vi "Histogram Window.vi"() -> ()   [LabVIEW 2019, in "Histogram Window.lvlib"]
uses:
  Histogram Window.lvlib
  Histogram Window Q Element v2.ctl
  Histogram Window Q Action v2.ctl
  Updated Plot Info.ctl
  Plot Style 3.ctl
  Fit Plot Request Information.ctl
  <vilib>/Utility/miscctls.llb/LVPointDoubleTypeDef.ctl
  Fit Models.ctl
  <vilib>/Utility/miscctls.llb/LVPoint32TypeDef.ctl
  Plot Histogram.ctl
  Fit Settings.ctl
  <vilib>/Analysis/6fits.llb/Curve Fitting Criteria.ctl
  Ramp Type.ctl
  XY Graph Add-Ons.lvlib
  Notebook.lvlib
  Rich Text Box.lvlib
  <vilib>/Analysis/NI_AALPro.lvlib
  Plot Editor.lvlib
panel:
  out "Histogram Graph TipStrip":string caption="Histogram TipStrip"
  out "Histogram Graph":cluster{"Axis":dbl[], "Histogram":dbl[]}[](graph)
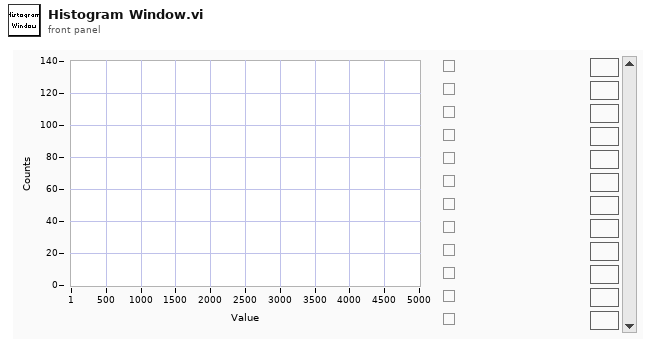
[diagram p1: front panel]
types:
  T1 = typedef "Histogram Window.lvlib/Histogram Window Q Element v2.ctl" = cluster{"Histogram Window Q Action":T2, "Data":variant}
  T2 = typedef "Histogram Window.lvlib/Histogram Window Q Action v2.ctl" = enum16{"Initialization", "Add Histogram", "Delete Histogram", "Delete Selected Histograms", "Clear Graph", "Change Bin Size", "Invert Histogram", "Update Graph", "Edit Plot", "Plot Fit", "Export XYGraph to Notebook", "Select All Plots", "Deselect All Plots", "Invert Plots Selection", "Set Style of Selected Plots", "Save Plot", "Save Selected Plots", "Save All Plots", "Quit"}
  T3 = cluster{"Event Registration Refnum":refnum<event-registration>}
  T4 = typedef "Histogram Window.lvlib/Updated Plot Info.ctl" = cluster{"Plot Index":i32, "Plot Name":string, "# Plots":i32, "Plot Style":T5}
  T5 = typedef "Plot Style 3.ctl" = cluster{"Plot Style":enum16{"unchanged", "Line", "Symbol", "Line + Symbol", "Histogram", "Histogram + Symbol"}, "Histogram Type":enum16{"unchanged", "Left Bound", "Center", "Right Bound"}, "Line Tickness":enum16{"unchanged", "Thin", "1 pixel", "2 pixel", "3 pixel", "4 pixel", "5 pixel"}, "Line Style":enum16{"unchanged", "Plain", "Long Dash", "Short Dash", "Long-Short Dash", "Long-Short-Short Dash"}, "Point Style":enum16{"unchanged", "None", "Empty Circle", "Filled Circle", "Thick Circle", "Dotted Circle", "Empty Square", "Filled Square", "Thick Square", "Dotted Square", "Small Filled Square", "Dot", "Cross", "Tiny Cross", "Large X", "Small x", "Diamond", "Small Empty Square"}, "Line Color":u32, "Point Color":u32, "Anti-aliased":bool, "Line Color Chooser":enum16{"unchanged", "Color Box", "Color List"}, "Point Color Chooser":enum16{"unchanged", "Color Box", "Color List"}, "Line Color List":string, "Point Color List":string}
  T6 = typedef "Histogram Window.lvlib/Plot Histogram.ctl" = cluster{"Plot Name":string, "Histogram":cluster{"Axis":dbl[], "Histogram":dbl[]}, "Plot Style":T5}
  T7 = typedef "LVPoint32TypeDef.ctl" = cluster{"Horizontal":i32, "Vertical":i32}
  T8 = typedef "Fit Plot Request Information.ctl" = cluster{"XY Graph Ref":refnum<vi>, "Mouse Coordinates":T9, "Fit Model":T10, "Plot Index":i32}
  T9 = typedef "LVPointDoubleTypeDef.ctl" = cluster{"X":dbl, "Y":dbl}
  T10 = typedef "Fit Models.ctl" = enum16{"Select a Fit Model...", "           Single Peak", "Gaussian", "Asymmetric Gaussian", "Lorentzian", "Asymmetric Lorentzian", "Gaussian/Lorentzian", "Lorentzian/Gaussian", "           Double Peak", "Two Gaussians", "Two Asymmetric Gaussians", "Two H-Connected Gaussians", "Two T-Connected Gaussians", "Two H-Connected Asymmetric Gaussians", "Two T-Connected Asymmetric Gaussians", "           Triple Peak", "Three Gaussians", "Three Asymmetric Gaussians", "              Decays", "Single Exponential", "Two Exponentials", "               ACF", "2D Gaussian ACF", "2D Gaussian + Blinking ACF", "2D Gaussian + Flow ACF", "3D Gaussian ACF", "3D Gaussian + Blinking ACF", "             Multiplot", "2D Gaussian ACF & 2D Gaussian + Flow ACF"}
  T11 = typedef "Fit Settings.ctl" = cluster{"Use Histogram # Points":bool, "# Fit Plot Points":u32, "Fit Method":T12, "Weighted Histogram Fit":bool, "Show All Fit Components":bool, "Ramp Type":T13}
  T12 = typedef "NI_AALPro.lvlib/Curve Fitting Criteria.ctl" = u16
  T13 = typedef "Ramp Type.ctl" = u16
  T14 = cluster{"CtlRef":refnum<vi>, "Select All Plots":bool}
  T15 = typedef "XY Graph Add-Ons.lvlib/XY Graph Refnum.ctl" = refnum<vi>
  T16 = typedef "D-Only Fixed Parameters.ctl" = cluster{"Fix D-only Peak Location":bool, "Peak Location":dbl, "Fix D-only Peak FWHM":bool, "Peak FWHM":dbl}
  T17 = typedef "Rich Text Box.lvlib/Text Formatting.ctl" = cluster{"Font":string, "Text Color":T18, "Text Background Color":T18, "Text Style":enum16{"Regular", "Bold", "Italic", "Underline", "Strikeout"}, "Font Size (Points)":dbl, "Text Alignment":i32}
  T18 = typedef "Rich Text Box.lvlib/Text Colors.ctl" = enum16{"Unchanged", "Black", "Blue", "Gray", "Green", "Red", "White"}
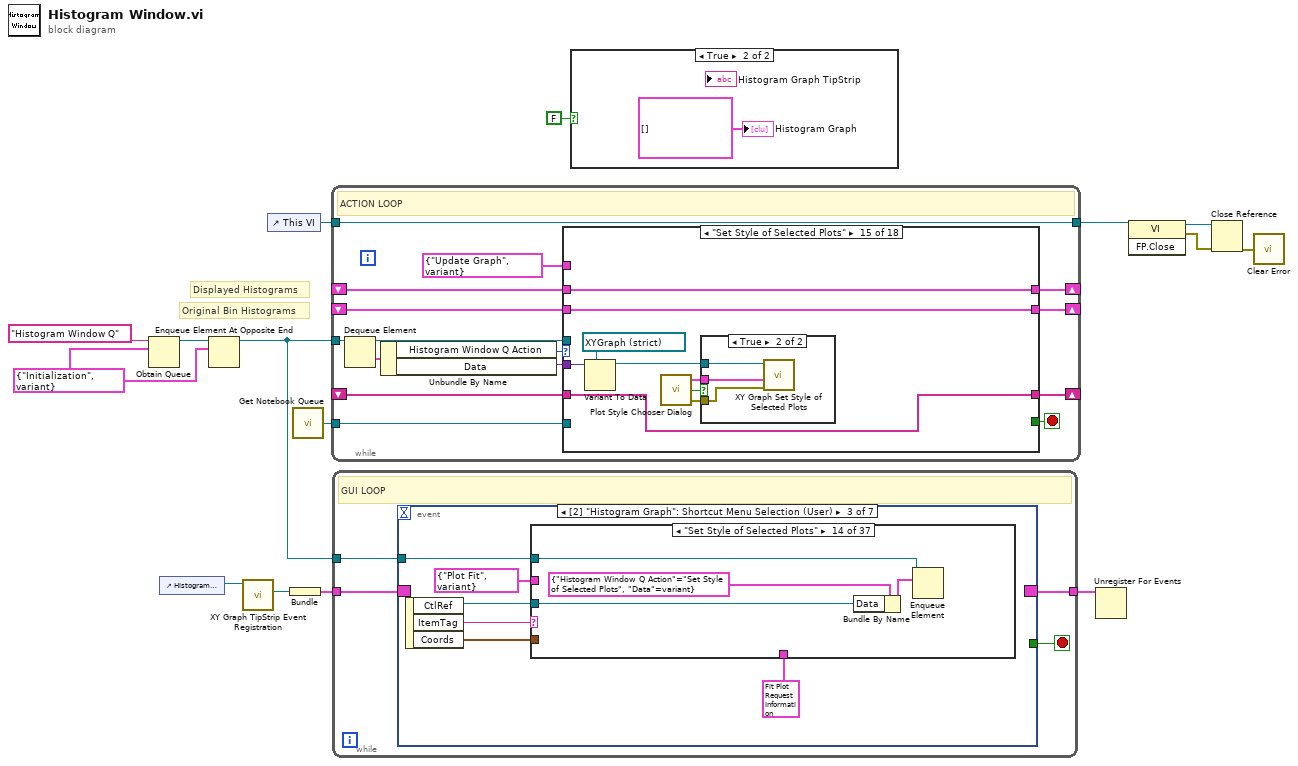
[diagram p0: block diagram]
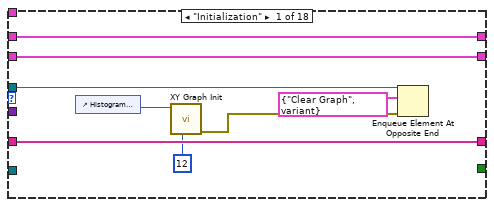
[diagram p3: hidden frame]
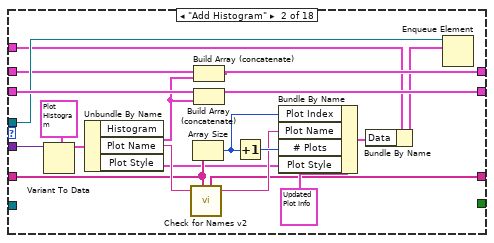
[diagram p4: hidden frame]
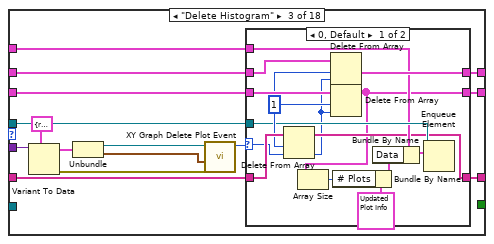
[diagram p5: hidden frame]
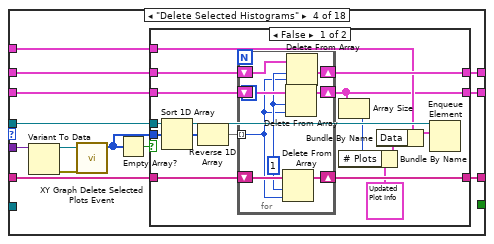
[diagram p7: hidden frame]
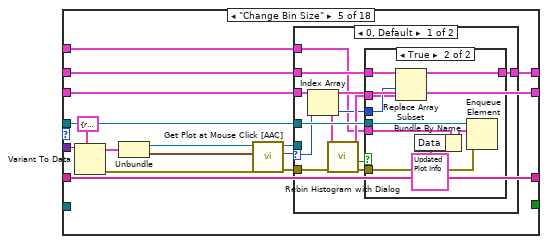
[diagram p9: hidden frame]
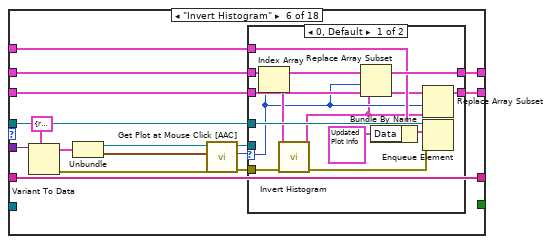
[diagram p12: hidden frame]
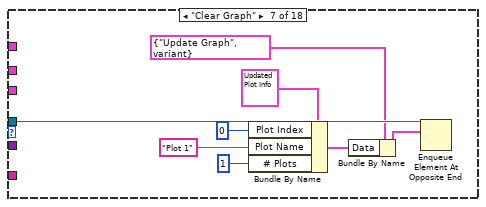
[diagram p14: hidden frame]
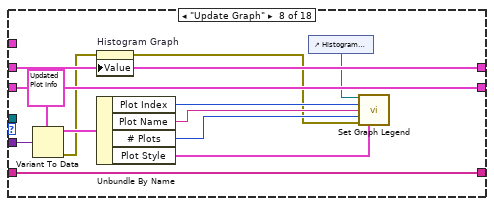
[diagram p15: hidden frame]
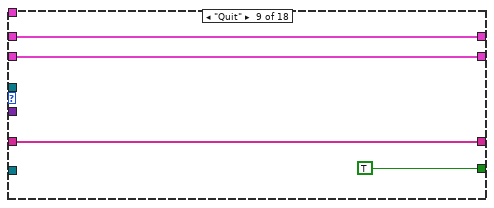
[diagram p16: hidden frame]
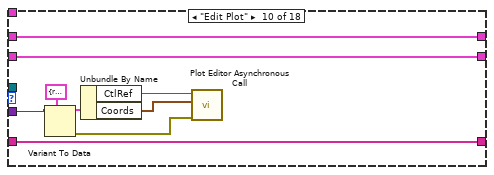
[diagram p17: hidden frame]
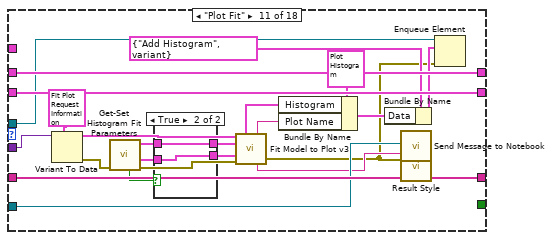
[diagram p18: hidden frame]
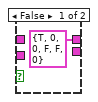
[diagram p19: hidden frame]
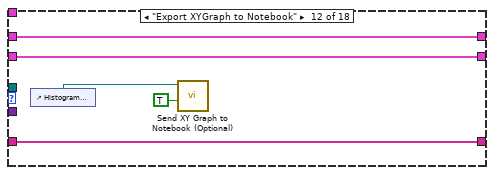
[diagram p20: hidden frame]
diagram:
  w10 = T1 {"Histogram Window Q Action"=enum."Initialization", "Data"=variant} ("ALEX TT Histogram Q Element")
  # "Displayed Histograms"
  # "Original Bin Histograms"
  n1 = Obtain Queue(name (unnamed)="Histogram Window Q", element data type=w10) -> (queue out=w14:refnum<queue>)  [unwired: 3 in, 2 out]
  n2 = control-ref of="Histogram Graph"() -> (w4:refnum<vi>)
  n3 = Enqueue Element At Opposite End(queue=w14, element=w10) -> (queue out=w11:refnum<queue>)  [unwired: 2 in, 2 out]
  n4 = call "XY Graph TipStrip Event Registration.vi"("XY Graph Refnum"=w4) -> ("Event Registration Refnum"=w3:refnum<event-registration>)  [unwired: 8 in, 2 out]
  n5 = control-ref of="This VI"() -> (w6:refnum<vi>)
  n6 = Bundle("Event Registration Refnum"=w3) -> (w8:T3)  [unwired: 1 in]
  n7 = call "Get Notebook Queue.vi"() -> ("Notebook Queue"=w9:refnum<queue>)  [unwired: 9 in]
  n8 = while {
    tunnel: w11 -> [w30]
    shift-right: [w24] -> _
    shift-left: _ -> [w25]
    shift-right: [w22] -> _
    shift-left: _ -> [w23]
    shift-right: [w19] -> _
    shift-left: _ -> [w20]
    tunnel: w9 -> [w17]
    tunnel: w6 -> [w16]
    tunnel: [w16] -> w5
    stop <- w27 stop-if-true
    # "ACTION LOOP"
    n9 = Dequeue Element(queue=w30) -> (queue out=w21:refnum<queue>, element=w29:T1)  [unwired: 2 in, 2 out]
    n10 = Unbundle By Name(w29) -> ("Histogram Window Q Action"=w28:T2, "Data"=w26:variant)
    n11 = case shown="\"Set Style of Selected Plots\"" w28 {
      tunnel: [_ _ _ _ _ _ _ _ TRUE _ _ _ _ _ _ _ _ _] -> w27
      tunnel: w26 -> [_ w57 w73 w103 w144 w182 _ w215 _ w223 w255 _ w266 w275 w282 w301 w313 w324]
      tunnel: w25 -> [w35 w40 w66 w100 w139 w177 _ w218 w219 w231 w247 w261 w272 w278 w279 w308 w319 w330]
      tunnel: [w35 w41 w65 w99 w139 w177 _ w218 w219 w231 w247 w261 w272 w278 w279 w308 w319 w330] -> w24
      tunnel: w23 -> [w36 w58 w68 w102 w133 w168 _ w217 w220 w230 w253 w262 w271 w277 w287 w307 w318 w329]
      tunnel: [w36 w54 w67 w101 w133 w167 _ w217 w220 w230 w253 w262 w271 w277 w287 w307 w318 w329] -> w22
      tunnel: w21 -> [w38 w52 w63 w98 w134 w172 w205 _ _ _ w252 _ _ _ _ _ _ _]
      tunnel: w20 -> [w37 w51 w62 w97 w132 w171 _ w216 w221 w229 w254 w263 w270 w276 w286 w306 w317 w328]
      tunnel: [w37 w49 w61 w96 w131 w170 _ w216 w221 w229 w254 w263 w270 w276 w286 w306 w317 w328] -> w19
      tunnel: T1 {"Histogram Window Q Action"=enum."Update Graph", "Data"=variant} ("ALEX TT Histogram Q Element") -> [_ w45 w60 w95 w130 w169 _ _ _ _ _ _ _ _ _ _ _ _]
      tunnel: w17 -> [_ _ _ _ _ _ _ _ _ _ w243 _ _ _ _ w299 w311 w322]
      frame "Initialization" {
        n12 = control-ref of="Histogram Graph"() -> (w31:refnum<vi>)
        n13 = call "XY Graph Init.vi"("Max Legend Size (8)"=12 ("32bit integer"), "XYGraph in"=w31) -> ("Error Out"=w33:errorcluster)  [unwired: 9 in]
        n14 = Enqueue Element At Opposite End(queue=w38, element=T1 {"Histogram Window Q Action"=enum."Clear Graph", "Data"=variant}, error in (no error)=w33) -> ()  [unwired: 1 in, 3 out]
      }
      frame "Add Histogram" {
        n15 = Variant To Data(type=T6 {"Plot Name"="", "Histogram"={"Axis"=[], "Histogram"=[]}, "Plot Style"={"Plot Style"=enum."Histogram + Symbol", "Histogram Type"=enum."Right Bound", "Line Tickness"=enum."unchanged", "Line Style"=enum."unchanged", "Point Style"=enum."unchanged", "Line Color"=0, "Point Color"=0, "Anti-aliased"=FALSE, "Line Color Chooser"=enum."unchanged", "Point Color Chooser"=enum."unchanged", "Line Color List"="", "Point Color List"=""}} ("output cluster"), Variant=w57) -> (data=w55:T6)  [unwired: 1 in, 1 out]
        n16 = Unbundle By Name(w55) -> ("Histogram"=w50:cluster{"Axis":dbl[], "Histogram":dbl[]}, "Plot Name"=w43:string, "Plot Style"=w39:T5)
        n17 = call "Check for Names v2.vi"("New Name"=w43, "Name List"=w40) -> ("New Name List"=w41:string[], "New Name"=w42:string)  [unwired: 4 in, 2 out]
        n18 = Array Size(array=w40) -> (size(s)=w48:i32)
        n19 = Build Array (concatenate)(w51, w50) -> (w49:cluster{"Axis":dbl[], "Histogram":dbl[]}[])
        n20 = Build Array (concatenate)(w58, w50) -> (w54:cluster{"Axis":dbl[], "Histogram":dbl[]}[])
        n21 = Increment(x=w48) -> (x+1=w53:i32)
        n22 = Bundle By Name(cluster=T4 {"Plot Index"=0, "Plot Name"="", "# Plots"=0, "Plot Style"={"Plot Style"=enum."Line + Symbol", "Histogram Type"=enum."Right Bound", "Line Tickness"=enum."Thin", "Line Style"=enum."unchanged", "Point Style"=enum."unchanged", "Line Color"=0, "Point Color"=0, "Anti-aliased"=FALSE, "Line Color Chooser"=enum."unchanged", "Point Color Chooser"=enum."unchanged", "Line Color List"="", "Point Color List"=""}} ("output cluster"), "Plot Index"=w48, "Plot Name"=w42, "# Plots"=w53, "Plot Style"=w39) -> (w46:T4)
        n23 = Bundle By Name(cluster=w45, "Data"=w46) -> (w47:T1)
        n24 = Enqueue Element(queue=w52, element=w47) -> ()  [unwired: 2 in, 3 out]
      }
      frame "Delete Histogram" {
        n25 = Variant To Data(type=cluster{"CtlRef":refnum<vi>, "Coords":T7} {"CtlRef"=refnum, "Coords"={"Horizontal"=0, "Vertical"=0}} ("output cluster"), Variant=w73) -> (data=w72:cluster{"CtlRef":refnum<vi>, "Coords":T7}, error out=w64:errorcluster)  [unwired: 1 in]
        n26 = Unbundle(w72) -> ("CtlRef"=w70:refnum<vi>, "Coords"=w69:T7)
        n27 = call "XY Graph Delete Plot Event.vi"("Error In"=w64, "Mouse Click Coordinates"=w69, "XYGraph Ref"=w70) -> ("Deleted Plot Index"=w59:i32)  [unwired: 4 in, 4 out]
        n28 = case shown="0, Default" w59 {
          selector: w59 -> [w76 _]
          tunnel: w68 -> [w87 w90]
          tunnel: [w74 w90] -> w67
          tunnel: w66 -> [w86 w89]
          tunnel: [w79 w89] -> w65
          tunnel: w63 -> [w82 _]
          tunnel: w62 -> [w85 w88]
          tunnel: [w84 w88] -> w61
          tunnel: w60 -> [w80 _]
          frame 0, Default {
            w83 = 1 ("length")
            n29 = Delete From Array(array=w86, length=w83, index=w76) -> (array with subset deleted=w79:string[])  [unwired: 1 out]
            n30 = Delete From Array(array=w85, length=w83, index=w76) -> (array with subset deleted=w84:cluster{"Axis":dbl[], "Histogram":dbl[]}[])  [unwired: 1 out]
            n31 = Delete From Array(array=w87, length=w83, index=w76) -> (array with subset deleted=w74:cluster{"Axis":dbl[], "Histogram":dbl[]}[])  [unwired: 1 out]
            n32 = Array Size(array=w74) -> (size(s)=w75:i32)
            n33 = Bundle By Name(cluster=T4 {"Plot Index"=-1, "Plot Name"="", "# Plots"=0, "Plot Style"={"Plot Style"=enum."Histogram + Symbol", "Histogram Type"=enum."Right Bound", "Line Tickness"=enum."unchanged", "Line Style"=enum."unchanged", "Point Style"=enum."unchanged", "Line Color"=0, "Point Color"=0, "Anti-aliased"=FALSE, "Line Color Chooser"=enum."unchanged", "Point Color Chooser"=enum."unchanged", "Line Color List"="", "Point Color List"=""}} ("output cluster"), "# Plots"=w75) -> (w78:T4)
            n34 = Bundle By Name(cluster=w80, "Data"=w78) -> (w81:T1)
            n35 = Enqueue Element(queue=w82, element=w81) -> ()  [unwired: 2 in, 3 out]
          }
          frame -1 {
          }
        }
      }
      frame "Delete Selected Histograms" {
        n36 = Variant To Data(Variant=w103) -> (data=w93:T15, error out=w94:errorcluster)  [unwired: 2 in]
        n37 = call "XY Graph Delete Selected Plots Event.vi"("Error In"=w94, "XYGraph Ref"=w93) -> ("Deleted Plot Indices"=w91:i32[])  [unwired: 5 in, 4 out]
        n38 = Empty Array?(array=w91) -> (empty?=w92:bool)
        n39 = case shown="False" w92 {
          tunnel: w102 -> [w118 w129]
          tunnel: [w107 w129] -> w101
          tunnel: w100 -> [w117 w128]
          tunnel: [w111 w128] -> w99
          tunnel: w98 -> [w114 _]
          tunnel: w97 -> [w116 w127]
          tunnel: [w115 w127] -> w96
          tunnel: w95 -> [w112 _]
          tunnel: w91 -> [w106 _]
          frame False {
            n40 = Sort 1D Array(array=w106) -> (sorted array=w105:i32[])
            n41 = Reverse 1D Array(array=w105) -> (reversed array=w104:i32[])
            n42 = for {
              shift-right: [w123] -> w115
              shift-left: w116 -> [w124]
              shift-right: [w120] -> w107
              shift-left: w118 -> [w126]
              shift-right: [w121] -> w111
              shift-left: w117 -> [w125]
              tunnel: w104 -> [w119] mode=indexing
              w122 = 1 ("length")
              n43 = Delete From Array(array=w125, length=w122, index=w119) -> (array with subset deleted=w121:string[])  [unwired: 1 out]
              n44 = Delete From Array(array=w126, length=w122, index=w119) -> (array with subset deleted=w120:cluster{"Axis":dbl[], "Histogram":dbl[]}[])  [unwired: 1 out]
              n45 = Delete From Array(array=w124, length=w122, index=w119) -> (array with subset deleted=w123:cluster{"Axis":dbl[], "Histogram":dbl[]}[])  [unwired: 1 out]
            }
            n46 = Array Size(array=w107) -> (size(s)=w108:i32)
            n47 = Bundle By Name(cluster=T4 {"Plot Index"=-1, "Plot Name"="", "# Plots"=0, "Plot Style"={"Plot Style"=enum."Histogram + Symbol", "Histogram Type"=enum."Right Bound", "Line Tickness"=enum."unchanged", "Line Style"=enum."unchanged", "Point Style"=enum."unchanged", "Line Color"=0, "Point Color"=0, "Anti-aliased"=FALSE, "Line Color Chooser"=enum."unchanged", "Point Color Chooser"=enum."unchanged", "Line Color List"="", "Point Color List"=""}} ("output cluster"), "# Plots"=w108) -> (w110:T4)
            n48 = Bundle By Name(cluster=w112, "Data"=w110) -> (w113:T1)
            n49 = Enqueue Element(queue=w114, element=w113) -> ()  [unwired: 2 in, 3 out]
          }
          frame True {
          }
        }
      }
      frame "Change Bin Size" {
        n50 = Variant To Data(type=cluster{"CtlRef":refnum<vi>, "Coords":T7} {"CtlRef"=refnum, "Coords"={"Horizontal"=0, "Vertical"=0}} ("output cluster"), Variant=w144) -> (data=w143:cluster{"CtlRef":refnum<vi>, "Coords":T7}, error out=w138:errorcluster)  [unwired: 1 in]
        n51 = Unbundle(w143) -> ("CtlRef"=w141:refnum<vi>, "Coords"=w140:T7)
        n52 = call "Get Plot at Mouse Click [AAC].vi"("error in (no error)"=w138, "Mouse Click Coordinates"=w140, "XYGraph Ref"=w141) -> ("error out"=w136:errorcluster, "Plot at Coordinates"=w137:i32, "XYGraph Ref"=w135:T15)  [unwired: 2 in, 4 out]
        n53 = case shown="0, Default" w137 {
          selector: w137 -> [w146 _]
          tunnel: w136 -> [w155 _]
          tunnel: w135 -> [_ _]
          tunnel: w134 -> [w154 _]
          tunnel: w133 -> [w152 _]
          tunnel: w132 -> [w149 w166]
          tunnel: [w148 w166] -> w131
          tunnel: w130 -> [w145 _]
          frame 0, Default {
            n54 = Index Array(array=w152, index=w146) -> (element=w151:cluster{"Axis":dbl[], "Histogram":dbl[]})
            n55 = call "Rebin Histogram with Dialog.vi"("error in (no error)"=w155, "Original Bin Histogram"=w151) -> ("error out"=w153:errorcluster, "OK?"=w150:bool, "Rebinned Histogram"=w147:cluster{"Axis":dbl[], "Histogram":dbl[]})  [unwired: 7 in]
            n56 = case shown="True" w150 {
              tunnel: w154 -> [_ w165]
              tunnel: w153 -> [_ w164]
              tunnel: w149 -> [w156 w163]
              tunnel: [w156 w162] -> w148
              tunnel: w147 -> [_ w160]
              tunnel: w146 -> [_ w161]
              tunnel: w145 -> [_ w159]
              frame False {
              }
              frame True {
                n57 = Replace Array Subset(array=w163, new element=w160, index=w161) -> (w162:cluster{"Axis":dbl[], "Histogram":dbl[]}[])
                n58 = Bundle By Name(cluster=w159, "Data"=T4 {"Plot Index"=-1, "Plot Name"="", "# Plots"=0, "Plot Style"={"Plot Style"=enum."Histogram + Symbol", "Histogram Type"=enum."Right Bound", "Line Tickness"=enum."unchanged", "Line Style"=enum."unchanged", "Point Style"=enum."unchanged", "Line Color"=0, "Point Color"=0, "Anti-aliased"=FALSE, "Line Color Chooser"=enum."unchanged", "Point Color Chooser"=enum."unchanged", "Line Color List"="", "Point Color List"=""}} ("Updated Plot Info")) -> (w158:T1)
                n59 = Enqueue Element(queue=w165, element=w158, error in (no error)=w164) -> ()  [unwired: 1 in, 3 out]
              }
            }
          }
          frame -1 {
          }
        }
      }
      frame "Invert Histogram" {
        n60 = Variant To Data(type=cluster{"CtlRef":refnum<vi>, "Coords":T7} {"CtlRef"=refnum, "Coords"={"Horizontal"=0, "Vertical"=0}} ("output cluster"), Variant=w182) -> (data=w181:cluster{"CtlRef":refnum<vi>, "Coords":T7}, error out=w176:errorcluster)  [unwired: 1 in]
        n61 = Unbundle(w181) -> ("CtlRef"=w179:refnum<vi>, "Coords"=w178:T7)
        n62 = call "Get Plot at Mouse Click [AAC].vi"("error in (no error)"=w176, "Mouse Click Coordinates"=w178, "XYGraph Ref"=w179) -> ("error out"=w174:errorcluster, "Plot at Coordinates"=w175:i32, "XYGraph Ref"=w173:T15)  [unwired: 2 in, 4 out]
        n63 = case shown="0, Default" w175 {
          selector: w175 -> [w185 _]
          tunnel: w174 -> [w195 _]
          tunnel: w173 -> [_ _]
          tunnel: w172 -> [w194 _]
          tunnel: w171 -> [w190 w197]
          tunnel: [w192 w197] -> w170
          tunnel: w169 -> [w191 _]
          tunnel: w168 -> [w186 w196]
          tunnel: [w183 w196] -> w167
          frame 0, Default {
            n64 = Index Array(array=w190, index=w185) -> (element=w189:cluster{"Axis":dbl[], "Histogram":dbl[]})
            n65 = call "Invert Histogram.vi"("error in (no error)"=w195, "Histogram"=w189) -> ("error out"=w193:errorcluster, "Inverted Histogram"=w184:cluster{"Axis":dbl[], "Histogram":dbl[]})  [unwired: 8 in]
            n66 = Replace Array Subset(array=w190, new element=w184, index=w185) -> (w192:cluster{"Axis":dbl[], "Histogram":dbl[]}[])
            n67 = Bundle By Name(cluster=w191, "Data"=T4 {"Plot Index"=-1, "Plot Name"="", "# Plots"=0, "Plot Style"={"Plot Style"=enum."Histogram + Symbol", "Histogram Type"=enum."Right Bound", "Line Tickness"=enum."unchanged", "Line Style"=enum."unchanged", "Point Style"=enum."unchanged", "Line Color"=0, "Point Color"=0, "Anti-aliased"=FALSE, "Line Color Chooser"=enum."unchanged", "Point Color Chooser"=enum."unchanged", "Line Color List"="", "Point Color List"=""}} ("output cluster")) -> (w188:T1)
            n68 = Replace Array Subset(array=w186, new element=w184, index=w185) -> (w183:cluster{"Axis":dbl[], "Histogram":dbl[]}[])
            n69 = Enqueue Element(queue=w194, element=w188, error in (no error)=w193) -> ()  [unwired: 1 in, 3 out]
          }
          frame -1 {
          }
        }
      }
      frame "Clear Graph" {
        n70 = Bundle By Name(cluster=T4 {"Plot Index"=0, "Plot Name"="", "# Plots"=0, "Plot Style"={"Plot Style"=enum."Histogram + Symbol", "Histogram Type"=enum."Right Bound", "Line Tickness"=enum."unchanged", "Line Style"=enum."unchanged", "Point Style"=enum."unchanged", "Line Color"=0, "Point Color"=0, "Anti-aliased"=FALSE, "Line Color Chooser"=enum."unchanged", "Point Color Chooser"=enum."unchanged", "Line Color List"="", "Point Color List"=""}} ("output cluster"), "Plot Index"=0, "Plot Name"="Plot 1", "# Plots"=1 ("# Legend Rows")) -> (w201:T4)
        n71 = Bundle By Name(cluster=T1 {"Histogram Window Q Action"=enum."Update Graph", "Data"=variant} ("ALEX TT Histogram Q Element"), "Data"=w201) -> (w203:T1)
        n72 = Enqueue Element At Opposite End(queue=w205, element=w203) -> ()  [unwired: 2 in, 3 out]
      }
      frame "Update Graph" {
        n73 = Variant To Data(type=T4 {"Plot Index"=0, "Plot Name"="", "# Plots"=0, "Plot Style"={"Plot Style"=enum."Histogram + Symbol", "Histogram Type"=enum."Right Bound", "Line Tickness"=enum."unchanged", "Line Style"=enum."unchanged", "Point Style"=enum."unchanged", "Line Color"=0, "Point Color"=0, "Anti-aliased"=FALSE, "Line Color Chooser"=enum."unchanged", "Point Color Chooser"=enum."unchanged", "Line Color List"="", "Point Color List"=""}} ("output cluster"), Variant=w215) -> (data=w213:T4, error out=w208:errorcluster)  [unwired: 1 in]
        n74 = property on="Histogram Graph" class="XYGraph (strict)"(error in=w208, "Value"=w216) -> (error out=w207:errorcluster)  [unwired: 1 in, 1 out]
        n75 = Unbundle By Name(w213) -> ("Plot Index"=w212:i32, "Plot Name"=w210:string, "# Plots"=w211:i32, "Plot Style"=w206:T5)
        n76 = control-ref of="Histogram Graph"() -> (w209:refnum<vi>)
        n77 = call "Set Graph Legend.vi"("XYGraph in"=w209, "Active Plot"=w212, "Plot Name"=w210, "# Plots"=w211, "error in (no error)"=w207, "Plot Style"=w206) -> ()  [unwired: 9 in, 1 out]
      }
      frame "Quit" {
      }
      frame "Edit Plot" {
        n78 = Variant To Data(type=cluster{"CtlRef":refnum<vi>, "Coords":T7} {"CtlRef"=refnum, "Coords"={"Horizontal"=0, "Vertical"=0}} ("output cluster"), Variant=w223) -> (data=w225:cluster{"CtlRef":refnum<vi>, "Coords":T7}, error out=w227:errorcluster)  [unwired: 1 in]
        n79 = Unbundle By Name(w225) -> ("CtlRef"=w228:refnum<vi>, "Coords"=w226:T7)
        n80 = call "Plot Editor Asynchronous Call.vi"("error in (no error)"=w227, "Coords"=w226, "XYGraph in"=w228) -> ()  [unwired: 5 in, 4 out]
      }
      frame "Plot Fit" {
        n81 = Variant To Data(type=T8 {"XY Graph Ref"=refnum, "Mouse Coordinates"={"X"=0.0, "Y"=0.0}, "Fit Model"=enum."Select a Fit Model...", "Plot Index"=-1} ("output cluster"), Variant=w255) -> (data=w240:T8, error out=w238:errorcluster)  [unwired: 1 in]
        n82 = call "Get-Set Histogram Fit Parameters.vi"("Error In"=w238) -> ("Error Out"=w237:errorcluster, "Fixed Parameters"=w232:T16, "Fit Settings"=w235:T11, "Initialized?"=w236:bool)  [unwired: 7 in]
        n83 = case shown="True" w236 {
          tunnel: w235 -> [_ w258]
          tunnel: [T11 {"Use Histogram # Points"=TRUE, "# Fit Plot Points"=0, "Fit Method"=0, "Weighted Histogram Fit"=FALSE, "Show All Fit Components"=FALSE, "Ramp Type"=0} ("Fit Settings") w258] -> w234
          tunnel: [_ w257] -> w233
          tunnel: w232 -> [_ w257]
          frame False {
          }
          frame True {
          }
        }
        n84 = call "Fit Model to Plot v3.vi"("Fit Plot Information"=w240, "Fit Settings"=w234, "Fixed Parameters"=w233, "error in (no error)"=w237) -> ("Fitted Plot"=w245:cluster{"X Array":dbl[], "Y Array":dbl[]}, "Plot Name"=w244:string, "Fit Result String"=w242:string, "error out"=w241:errorcluster)  [unwired: 5 in, 3 out]
        n85 = Bundle By Name(cluster=T6 {"Plot Name"="", "Histogram"={"Axis"=[], "Histogram"=[]}, "Plot Style"={"Plot Style"=enum."Line", "Histogram Type"=enum."Center", "Line Tickness"=enum."2 pixel", "Line Style"=enum."Plain", "Point Style"=enum."None", "Line Color"=16711680, "Point Color"=16711680, "Anti-aliased"=TRUE, "Line Color Chooser"=enum."Color Box", "Point Color Chooser"=enum."Color Box", "Line Color List"="", "Point Color List"=""}} ("output cluster"), "Histogram"=w245, "Plot Name"=w244) -> (w249:T6)
        n86 = Bundle By Name(cluster=T1 {"Histogram Window Q Action"=enum."Add Histogram", "Data"=variant} ("element"), "Data"=w249) -> (w250:T1)
        n87 = call "Result Style.vi"() -> ("Default Text Formatting"=w239:T17)
        n88 = call "Send Message to Notebook.vi"("Notebook Queue"=w243, "Message"=w242, "Error In"=w241, "Text Formatting"=w239) -> ()  [unwired: 15 in, 1 out]
        n89 = Enqueue Element(queue=w252, element=w250, error in (no error)=w241) -> ()  [unwired: 1 in, 3 out]
      }
      frame "Export XYGraph to Notebook" {
        n90 = control-ref of="Histogram Graph"() -> (w260:refnum<vi>)
        n91 = call "Send XY Graph to Notebook (Optional).vi"("Send Graph to Notebook?"=TRUE, "XYGraph in"=w260) -> ()  [unwired: 9 in, 1 out]
      }
      frame "Select All Plots", "Deselect All Plots" {
        n92 = Variant To Data(type=T14 {"CtlRef"=refnum, "Select All Plots"=TRUE} ("output cluster"), Variant=w266) -> (data=w269:T14, error out=w264:errorcluster)  [unwired: 1 in]
        n93 = Unbundle(w269) -> ("CtlRef"=w268:refnum<vi>, "Select All Plots"=w267:bool)
        n94 = call "XY Graph Select All Plots Event.vi"("Error In"=w264, "Select (T)/Deselect"=w267, "XYGraph Ref"=w268) -> ()  [unwired: 5 in, 4 out]
      }
      frame "Invert Plots Selection" {
        n95 = Variant To Data(Variant=w275) -> (data=w274:T15, error out=w273:errorcluster)  [unwired: 2 in]
        n96 = call "XY Graph Invert Plots Selection Event.vi"("Error In"=w273, "XYGraph Ref"=w274) -> ()  [unwired: 6 in, 4 out]
      }
      frame "Set Style of Selected Plots" {
        n97 = Variant To Data(type=refnum<vi> refnum ("XYGraph Ref"), Variant=w282) -> (data=w280:refnum<vi>)  [unwired: 1 in, 1 out]
        n98 = call "Plot Style Chooser Dialog.vi"() -> ("Plot Style out"=w285:T5, "Cancelled?"=w284:bool, "Error Out"=w283:errorcluster)  [unwired: 7 in]
        n99 = case shown="True" w284 {
          tunnel: w280 -> [_ w290]
          tunnel: w285 -> [_ w289]
          tunnel: w283 -> [_ w288]
          frame False {
          }
          frame True {
            n100 = call "XY Graph Set Style of Selected Plots.vi"("Error In"=w288, "Plot Style"=w289, "XYGraph Ref"=w290) -> ()  [unwired: 5 in, 4 out]
          }
        }
      }
      frame "Save Plot" {
        n101 = Variant To Data(type=cluster{"CtlRef":refnum<vi>, "Coords":T7} {"CtlRef"=refnum, "Coords"={"Horizontal"=0, "Vertical"=0}} ("output cluster"), Variant=w301) -> (data=w304:cluster{"CtlRef":refnum<vi>, "Coords":T7}, error out=w300:errorcluster)  [unwired: 1 in]
        n102 = Unbundle By Name(w304) -> ("CtlRef"=w302:refnum<vi>, "Coords"=w303:T7)
        n103 = call "XY Graph Save Plot Event.vi"("Error In"=w300, "Mouse Click Coordinates"=w303, "XYGraph Ref"=w302) -> ("Error Out"=w294:errorcluster, "Message"=w297:string, "File Path"=w291:path, "Plot Name"=w292:string)  [unwired: 3 in, 2 out]
        n104 = Format Into String(format string=" from %s saved as %s", initial string=w297, error in=w294, w292, w291) -> (resulting string=w295:string, error out=w293:errorcluster)
        n105 = call "Message Style.vi"() -> ("Message Formatting"=w298:T17)
        n106 = call "Send Message to Notebook.vi"("Notebook Queue"=w299, "Message"=w295, "Error In"=w293, "Text Formatting"=w298) -> ()  [unwired: 15 in, 1 out]
      }
      frame "Save Selected Plots" {
        n107 = Variant To Data(Variant=w313) -> (data=w316:T15, error out=w314:errorcluster)  [unwired: 2 in]
        n108 = call "XY Graph Save Selected Plots Event.vi"("Error In"=w314, "Save All Plots? (T)"=FALSE, "XYGraph Ref"=w316) -> ("Error Out"=w310:errorcluster, "Message"=w309:string)  [unwired: 3 in, 4 out]
        n109 = call "Message Style.vi"() -> ("Message Formatting"=w312:T17)
        n110 = call "Send Message to Notebook.vi"("Notebook Queue"=w311, "Message"=w309, "Error In"=w310, "Text Formatting"=w312) -> ()  [unwired: 15 in, 1 out]
      }
      frame "Save All Plots" {
        n111 = Variant To Data(Variant=w324) -> (data=w327:T15, error out=w325:errorcluster)  [unwired: 2 in]
        n112 = call "XY Graph Save Selected Plots Event.vi"("Error In"=w325, "Save All Plots? (T)"=TRUE, "XYGraph Ref"=w327) -> ("Error Out"=w321:errorcluster, "Message"=w320:string)  [unwired: 3 in, 4 out]
        n113 = call "Message Style.vi"() -> ("Message Formatting"=w323:T17)
        n114 = call "Send Message to Notebook.vi"("Notebook Queue"=w322, "Message"=w320, "Error In"=w321, "Text Formatting"=w323) -> ()  [unwired: 15 in, 1 out]
      }
    }
  }
  n115 = while {
    tunnel: w11 -> [w333]
    tunnel: w8 -> [w331]
    tunnel: [w332] -> w2
    stop <- w334 stop-if-true
    # "GUI LOOP"
    n116 = event shown="[2] \"Histogram Graph\": Shortcut Menu Selection (User)" {
      selector: w331 -> [_ _ _ _ w557 w562 w563]
      dyn-events: [_ _ _ _ w556 w561 w563] -> w332
      timeout: _ -> [_ _ _ _ _ _ _]
      tunnel: [w337 _ _ _ _ _ _] -> w334
      tunnel: w333 -> [w336 w344 w347 _ _ _ _]
      event Panel Close? {
        w337 = TRUE
        n117 = event-data() -> ()  [unwired: 1 in, 3 out]
        n118 = Enqueue Element(queue=w336, element=T1 {"Histogram Window Q Action"=enum."Quit", "Data"=variant} ("ALEX TT Histogram Q Element")) -> ()  [unwired: 2 in, 3 out]
        n119 = event-data("Discard?"=w337) -> ()  [unwired: 1 in, 1 out]
      }
      event Pane Size {
        n120 = event-data() -> ()  [unwired: 1 in, 1 out]
        n121 = control-ref of="Histogram Graph"() -> (w339:refnum<vi>)
        n122 = call "XY Graph Number of Plots.vi"("XYGraph in"=w339) -> ("# Plots"=w338:i32)  [unwired: 9 in, 1 out]
        n123 = Bundle By Name(cluster=T4 {"Plot Index"=-1, "Plot Name"="", "# Plots"=0, "Plot Style"={"Plot Style"=enum."Histogram + Symbol", "Histogram Type"=enum."Right Bound", "Line Tickness"=enum."unchanged", "Line Style"=enum."unchanged", "Point Style"=enum."unchanged", "Line Color"=0, "Point Color"=0, "Anti-aliased"=FALSE, "Line Color Chooser"=enum."unchanged", "Point Color Chooser"=enum."unchanged", "Line Color List"="", "Point Color List"=""}} ("Updated Plot Info"), "# Plots"=w338) -> (w340:T4)
        n124 = Bundle By Name(cluster=T1 {"Histogram Window Q Action"=enum."Update Graph", "Data"=variant} ("element"), "Data"=w340) -> (w342:T1)
        n125 = Enqueue Element(queue=w344, element=w342) -> ()  [unwired: 2 in, 3 out]
      }
      event "Histogram Graph": Shortcut Menu Selection (User) {
        n126 = event-data() -> ("CtlRef"=w350:refnum<vi>, "ItemTag"=w349:string, "Coords"=w348:T7)  [unwired: 1 in]
        n127 = case shown="\"Set Style of Selected Plots\"" w349 {
          tunnel: w350 -> [_ w353 _ _ w362 w364 w372 w378 w384 w386 w394 w396 w404 w406 w410 w414 _ w424 w432 w440 w448 w456 w464 w472 w480 w488 w496 w504 w512 w520 w528 w536 w544 _ _ w548 w549]
          tunnel: w348 -> [_ w352 _ _ w361 _ w371 w377 w383 _ _ _ _ _ _ _ _ w423 w431 w439 w447 w455 w463 w471 w479 w487 w495 w503 w511 w519 w527 w535 w543 _ _ _ _]
          tunnel: w347 -> [_ w357 _ _ w363 w367 w373 w379 w385 w389 w395 w399 w405 w409 w413 w417 _ w425 w433 w441 w449 w457 w465 w473 w481 w489 w497 w505 w513 w521 w529 w537 w545 w547 _ _ _]
          tunnel: T1 {"Histogram Window Q Action"=enum."Plot Fit", "Data"=variant} ("ALEX TT Histogram Q Element") -> [_ _ _ _ _ _ _ _ _ _ _ _ _ _ _ _ _ w420 w427 w435 w443 w451 w459 w467 w475 w483 w491 w499 w507 w515 w523 w531 w540 _ _ _ _]
          tunnel: T8 {"XY Graph Ref"=refnum, "Mouse Coordinates"={"X"=0.0, "Y"=0.0}, "Fit Model"=enum."Select a Fit Model...", "Plot Index"=-1} ("output cluster") -> [_ _ _ _ _ _ _ _ _ _ _ _ _ _ _ _ _ w418 w426 w434 w442 w450 w458 w466 w474 w482 w490 w498 w506 w514 w522 w530 w539 _ _ _ _]
          frame "", Default {
          }
          frame "Edit Plot" {
            n128 = Bundle By Name(cluster=cluster{"CtlRef":refnum<vi>, "Coords":T7} {"CtlRef"=refnum, "Coords"={"Horizontal"=0, "Vertical"=0}} ("output cluster"), "CtlRef"=w353, "Coords"=w352) -> (w355:cluster{"CtlRef":refnum<vi>, "Coords":T7})
            n129 = Bundle By Name(cluster=T1 {"Histogram Window Q Action"=enum."Edit Plot", "Data"=variant} ("ALEX TT Histogram Q Element"), "Data"=w355) -> (w351:T1)
            n130 = Enqueue Element(queue=w357, element=w351) -> ()  [unwired: 2 in, 3 out]
          }
          frame "Send Plot to Advanced Plot Window" {
          }
          frame "Send Graph to Advanced Plot Window" {
          }
          frame "Delete Plot" {
            n131 = Bundle("CtlRef"=w362, "Coords"=w361) -> (w359:cluster{"CtlRef":refnum<vi>, "Coords":T7})  [unwired: 1 in]
            n132 = Bundle By Name(cluster=T1 {"Histogram Window Q Action"=enum."Delete Histogram", "Data"=variant} ("ALEX TT Histogram Q Element"), "Data"=w359) -> (w360:T1)
            n133 = Enqueue Element(queue=w363, element=w360) -> ()  [unwired: 2 in, 3 out]
          }
          frame "Delete Selected Plots" {
            n134 = Bundle By Name(cluster=T1 {"Histogram Window Q Action"=enum."Delete Selected Histograms", "Data"=variant} ("ALEX TT Histogram Q Element"), "Data"=w364) -> (w366:T1)
            n135 = Enqueue Element(queue=w367, element=w366) -> ()  [unwired: 2 in, 3 out]
          }
          frame "Save Plot" {
            n136 = Bundle("CtlRef"=w372, "Coords"=w371) -> (w369:cluster{"CtlRef":refnum<vi>, "Coords":T7})  [unwired: 1 in]
            n137 = Bundle By Name(cluster=T1 {"Histogram Window Q Action"=enum."Save Plot", "Data"=variant} ("ALEX TT Histogram Q Element"), "Data"=w369) -> (w370:T1)
            n138 = Enqueue Element(queue=w373, element=w370) -> ()  [unwired: 2 in, 3 out]
          }
          frame "Rebin Histogram" {
            n139 = Bundle("CtlRef"=w378, "Coords"=w377) -> (w375:cluster{"CtlRef":refnum<vi>, "Coords":T7})  [unwired: 1 in]
            n140 = Bundle By Name(cluster=T1 {"Histogram Window Q Action"=enum."Change Bin Size", "Data"=variant} ("ALEX TT Histogram Q Element"), "Data"=w375) -> (w376:T1)
            n141 = Enqueue Element(queue=w379, element=w376) -> ()  [unwired: 2 in, 3 out]
          }
          frame "Invert Histogram" {
            n142 = Bundle("CtlRef"=w384, "Coords"=w383) -> (w381:cluster{"CtlRef":refnum<vi>, "Coords":T7})  [unwired: 1 in]
            n143 = Bundle By Name(cluster=T1 {"Histogram Window Q Action"=enum."Invert Histogram", "Data"=variant} ("ALEX TT Histogram Q Element"), "Data"=w381) -> (w382:T1)
            n144 = Enqueue Element(queue=w385, element=w382) -> ()  [unwired: 2 in, 3 out]
          }
          frame "Clear Graph" {
            n145 = Bundle By Name(cluster=T1 {"Histogram Window Q Action"=enum."Clear Graph", "Data"=variant} ("ALEX TT Histogram Q Element"), "Data"=w386) -> (w388:T1)
            n146 = Enqueue Element(queue=w389, element=w388) -> ()  [unwired: 2 in, 3 out]
          }
          frame "Select All Plots" {
            n147 = Bundle("CtlRef"=w394, TRUE) -> (w392:cluster{"CtlRef":refnum<vi>, bool})  [unwired: 1 in]
            n148 = Bundle By Name(cluster=T1 {"Histogram Window Q Action"=enum."Select All Plots", "Data"=variant} ("ALEX TT Histogram Q Element"), "Data"=w392) -> (w393:T1)
            n149 = Enqueue Element(queue=w395, element=w393) -> ()  [unwired: 2 in, 3 out]
          }
          frame "Invert Plots Selection" {
            n150 = Bundle By Name(cluster=T1 {"Histogram Window Q Action"=enum."Invert Plots Selection", "Data"=variant} ("element"), "Data"=w396) -> (w397:T1)
            n151 = Enqueue Element(queue=w399, element=w397) -> ()  [unwired: 2 in, 3 out]
          }
          frame "Deselect All Plots" {
            n152 = Bundle("CtlRef"=w404, FALSE) -> (w402:cluster{"CtlRef":refnum<vi>, bool})  [unwired: 1 in]
            n153 = Bundle By Name(cluster=T1 {"Histogram Window Q Action"=enum."Select All Plots", "Data"=variant} ("ALEX TT Histogram Q Element"), "Data"=w402) -> (w403:T1)
            n154 = Enqueue Element(queue=w405, element=w403) -> ()  [unwired: 2 in, 3 out]
          }
          frame "Set Style of Selected Plots" {
            n155 = Bundle By Name(cluster=T1 {"Histogram Window Q Action"=enum."Set Style of Selected Plots", "Data"=variant} ("ALEX TT Histogram Q Element"), "Data"=w406) -> (w408:T1)
            n156 = Enqueue Element(queue=w409, element=w408) -> ()  [unwired: 2 in, 3 out]
          }
          frame "Save Selected Plots" {
            n157 = Bundle By Name(cluster=T1 {"Histogram Window Q Action"=enum."Save Selected Plots", "Data"=variant} ("ALEX TT Histogram Q Element"), "Data"=w410) -> (w412:T1)
            n158 = Enqueue Element(queue=w413, element=w412) -> ()  [unwired: 2 in, 3 out]
          }
          frame "Save All Plots" {
            n159 = Bundle By Name(cluster=T1 {"Histogram Window Q Action"=enum."Save All Plots", "Data"=variant} ("ALEX TT Histogram Q Element"), "Data"=w414) -> (w416:T1)
            n160 = Enqueue Element(queue=w417, element=w416) -> ()  [unwired: 2 in, 3 out]
          }
          frame "----------- Fits -----------" {
          }
          frame "Gaussian" {
            n161 = Bundle By Name(cluster=w418, "XY Graph Ref"=w424, "Mouse Coordinates"=w423, "Fit Model"=Fit_Models."Gaussian") -> (w422:T8)
            n162 = Bundle By Name(cluster=w420, "Data"=w422) -> (w419:T1)
            n163 = Enqueue Element(queue=w425, element=w419) -> ()  [unwired: 2 in, 3 out]
          }
          frame "Lorentzian" {
            n164 = Bundle By Name(cluster=w426, "XY Graph Ref"=w432, "Mouse Coordinates"=w431, "Fit Model"=Fit_Models."Lorentzian") -> (w429:T8)
            n165 = Bundle By Name(cluster=w427, "Data"=w429) -> (w430:T1)
            n166 = Enqueue Element(queue=w433, element=w430) -> ()  [unwired: 2 in, 3 out]
          }
          frame "Asymmetric Gaussian" {
            n167 = Bundle By Name(cluster=w434, "XY Graph Ref"=w440, "Mouse Coordinates"=w439, "Fit Model"=Fit_Models."Asymmetric Gaussian") -> (w437:T8)
            n168 = Bundle By Name(cluster=w435, "Data"=w437) -> (w438:T1)
            n169 = Enqueue Element(queue=w441, element=w438) -> ()  [unwired: 2 in, 3 out]
          }
          frame "Asymmetric Lorentzian" {
            n170 = Bundle By Name(cluster=w442, "XY Graph Ref"=w448, "Mouse Coordinates"=w447, "Fit Model"=Fit_Models."Asymmetric Lorentzian") -> (w445:T8)
            n171 = Bundle By Name(cluster=w443, "Data"=w445) -> (w446:T1)
            n172 = Enqueue Element(queue=w449, element=w446) -> ()  [unwired: 2 in, 3 out]
          }
          frame "Gaussian/Lorentzian" {
            n173 = Bundle By Name(cluster=w450, "XY Graph Ref"=w456, "Mouse Coordinates"=w455, "Fit Model"=Fit_Models."Gaussian/Lorentzian") -> (w453:T8)
            n174 = Bundle By Name(cluster=w451, "Data"=w453) -> (w454:T1)
            n175 = Enqueue Element(queue=w457, element=w454) -> ()  [unwired: 2 in, 3 out]
          }
          frame "Lorentzian/Gaussian" {
            n176 = Bundle By Name(cluster=w458, "XY Graph Ref"=w464, "Mouse Coordinates"=w463, "Fit Model"=Fit_Models."Lorentzian/Gaussian") -> (w461:T8)
            n177 = Bundle By Name(cluster=w459, "Data"=w461) -> (w462:T1)
            n178 = Enqueue Element(queue=w465, element=w462) -> ()  [unwired: 2 in, 3 out]
          }
          frame "1-Exponential" {
            n179 = Bundle By Name(cluster=w466, "XY Graph Ref"=w472, "Mouse Coordinates"=w471, "Fit Model"=Fit_Models."Single Exponential") -> (w469:T8)
            n180 = Bundle By Name(cluster=w467, "Data"=w469) -> (w470:T1)
            n181 = Enqueue Element(queue=w473, element=w470) -> ()  [unwired: 2 in, 3 out]
          }
          frame "2-Exponentials" {
            n182 = Bundle By Name(cluster=w474, "XY Graph Ref"=w480, "Mouse Coordinates"=w479, "Fit Model"=Fit_Models."Two Exponentials") -> (w477:T8)
            n183 = Bundle By Name(cluster=w475, "Data"=w477) -> (w478:T1)
            n184 = Enqueue Element(queue=w481, element=w478) -> ()  [unwired: 2 in, 3 out]
          }
          frame "Two Gaussians" {
            n185 = Bundle By Name(cluster=w482, "XY Graph Ref"=w488, "Mouse Coordinates"=w487, "Fit Model"=Fit_Models."Two Gaussians") -> (w485:T8)
            n186 = Bundle By Name(cluster=w483, "Data"=w485) -> (w486:T1)
            n187 = Enqueue Element(queue=w489, element=w486) -> ()  [unwired: 2 in, 3 out]
          }
          frame "Two Asymmetric Gaussians" {
            n188 = Bundle By Name(cluster=w490, "XY Graph Ref"=w496, "Mouse Coordinates"=w495, "Fit Model"=Fit_Models."Two Asymmetric Gaussians") -> (w493:T8)
            n189 = Bundle By Name(cluster=w491, "Data"=w493) -> (w494:T1)
            n190 = Enqueue Element(queue=w497, element=w494) -> ()  [unwired: 2 in, 3 out]
          }
          frame "Two H-Connected Gaussians" {
            n191 = Bundle By Name(cluster=w498, "XY Graph Ref"=w504, "Mouse Coordinates"=w503, "Fit Model"=Fit_Models."Two H-Connected Gaussians") -> (w501:T8)
            n192 = Bundle By Name(cluster=w499, "Data"=w501) -> (w502:T1)
            n193 = Enqueue Element(queue=w505, element=w502) -> ()  [unwired: 2 in, 3 out]
          }
          frame "Two T-Connected Gaussians" {
            n194 = Bundle By Name(cluster=w506, "XY Graph Ref"=w512, "Mouse Coordinates"=w511, "Fit Model"=Fit_Models."Two T-Connected Gaussians") -> (w509:T8)
            n195 = Bundle By Name(cluster=w507, "Data"=w509) -> (w510:T1)
            n196 = Enqueue Element(queue=w513, element=w510) -> ()  [unwired: 2 in, 3 out]
          }
          frame "Two H-Connected Asymmetric Gaussians" {
            n197 = Bundle By Name(cluster=w514, "XY Graph Ref"=w520, "Mouse Coordinates"=w519, "Fit Model"=Fit_Models."Two H-Connected Asymmetric Gaussians") -> (w517:T8)
            n198 = Bundle By Name(cluster=w515, "Data"=w517) -> (w518:T1)
            n199 = Enqueue Element(queue=w521, element=w518) -> ()  [unwired: 2 in, 3 out]
          }
          frame "Two T-Connected Asymmetric Gaussians" {
            n200 = Bundle By Name(cluster=w522, "XY Graph Ref"=w528, "Mouse Coordinates"=w527, "Fit Model"=Fit_Models."Two T-Connected Asymmetric Gaussians") -> (w525:T8)
            n201 = Bundle By Name(cluster=w523, "Data"=w525) -> (w526:T1)
            n202 = Enqueue Element(queue=w529, element=w526) -> ()  [unwired: 2 in, 3 out]
          }
          frame "Three Gaussians" {
            n203 = Bundle By Name(cluster=w530, "XY Graph Ref"=w536, "Mouse Coordinates"=w535, "Fit Model"=Fit_Models."Three Gaussians") -> (w533:T8)
            n204 = Bundle By Name(cluster=w531, "Data"=w533) -> (w534:T1)
            n205 = Enqueue Element(queue=w537, element=w534) -> ()  [unwired: 2 in, 3 out]
          }
          frame "Three Asymmetric Gaussians" {
            n206 = Bundle By Name(cluster=w539, "XY Graph Ref"=w544, "Mouse Coordinates"=w543, "Fit Model"=Fit_Models."Three Asymmetric Gaussians") -> (w541:T8)
            n207 = Bundle By Name(cluster=w540, "Data"=w541) -> (w542:T1)
            n208 = Enqueue Element(queue=w545, element=w542) -> ()  [unwired: 2 in, 3 out]
          }
          frame "Export Image to Notebook" {
            n209 = Enqueue Element(queue=w547, element=T1 {"Histogram Window Q Action"=enum."Export XYGraph to Notebook", "Data"=variant}) -> ()  [unwired: 2 in, 3 out]
          }
          frame "-------------" {
          }
          frame "Show/Hide Grid" {
            n210 = call "XY Graph Show-Hide Grid Event.vi"("XYGraph in"=w548) -> ()  [unwired: 9 in, 2 out]
          }
          frame "Show/Hide Tool Panels" {
            n211 = call "XY Graph Show-Hide Tool Panels Event.vi"("XYGraph in"=w549) -> ()  [unwired: 9 in, 2 out]
          }
        }
      }
      event "Histogram Graph": Shortcut Menu Activation? {
        n212 = event-data() -> ("CtlRef"=w552:refnum<vi>, "MenuRef"=w551:refnum<k9>)  [unwired: 1 in]
        n213 = call "XY Graph Check-Uncheck Menu Items.vi"("Menu in"=w551, "XY Graph Refnum"=w552) -> ()  [unwired: 8 in, 2 out]
        n214 = event-data("Discard?"=FALSE) -> ()  [unwired: 1 in, 1 out]
      }
      event Mouse Enter {
        n215 = event-data() -> ("CtlRef"=w555:refnum<vi>)  [unwired: 1 in]
        n216 = Unbundle By Name(w557) -> ("Event Registration Refnum"=w554:refnum<event-registration>)
        n217 = call "XY Graph Tipstrip Mouse Enter.vi"("Event Registration Refnum"=w554, "XY Graph Refnum"=w555) -> ("Event Registration Refnum"=w553:refnum<event-registration>)  [unwired: 8 in, 1 out]
        n218 = Bundle By Name(cluster=w557, "Event Registration Refnum"=w553) -> (w556:T3)
      }
      event Mouse Leave {
        n219 = event-data() -> ("CtlRef"=w560:refnum<vi>)  [unwired: 1 in]
        n220 = Unbundle By Name(w562) -> ("Event Registration Refnum"=w559:refnum<event-registration>)
        n221 = call "XY Graph Tipstrip Mouse Leave.vi"("Event Registration Refnum"=w559, "XY Graph Refnum"=w560) -> ("Event Registration Refnum"=w558:refnum<event-registration>)  [unwired: 8 in, 1 out]
        n222 = Bundle By Name(cluster=w562, "Event Registration Refnum"=w558) -> (w561:T3)
      }
      event Mouse Move {
        n223 = event-data() -> ("CtlRef"=w565:refnum<vi>, "Coords"=w564:T7)  [unwired: 1 in]
        n224 = call "XY Graph TipStrip Mouse Move.vi"("Coords"=w564, "XY Graph Refnum"=w565) -> ()  [unwired: 7 in, 3 out]
      }
    }
  }
  n225 = case shown="True" FALSE {
    frame False {
    }
    frame True {
      "Histogram Graph" <- cluster{"Axis":dbl[], "Histogram":dbl[]}[] [] ("Histogram Graph")
    }
  }
  n226 = Unregister For Events(event registration refnum=w2) -> ()  [unwired: 1 in, 1 out]
  n227 = invoke class="VI" method="FP.Close"(reference=w5) -> (reference out=w13:refnum<vi>, error out=w12:errorcluster)  [unwired: 2 in, 1 out]
  n228 = Close Reference(reference=w13, error in (no error)=w12) -> (error out=w1:errorcluster)
  n229 = call "Clear Error.vi"("Error In"=w1) -> ()  [unwired: 8 in, 1 out]
